vi "Periodic Tasks.vi"(8 "error in":errorcluster) -> ()   [LabVIEW 2017]
doc: "This VI runs in parallel to other tasks. It can contain as many user-defined periodic loops as you need. These can carry out PID or other sorts of timed response."
uses:
  <vilib>/Rock Robotics/WPI/ThirdParty/Phoenix-LabVIEW/Motor Controller/Controls/CTRE_Phoenix_MotorControl_ControlMode.ctl
  <vilib>/Rock Robotics/WPI/ThirdParty/Phoenix-LabVIEW/Motor Controller/Controls/CTRE_Phoenix_MotorControl_RemoteFeedbackDevice.ctl
  <vilib>/Rock Robotics/WPI/ThirdParty/Phoenix-LabVIEW/Motor Controller/Controls/CTRE_Phoenix_MotorControl_RemoteSourceType.ctl
  <vilib>/Rock Robotics/WPI/ThirdParty/Phoenix-LabVIEW/Controls/CTRE_Phoenix_Params.ctl
  <vilib>/Rock Robotics/WPI/Utilities/WPI_GetSetVariantRefNum.vi
panel:
  in  "Reverse Limit Threshold":i32
  in  "Forward Limit Threshold":i32
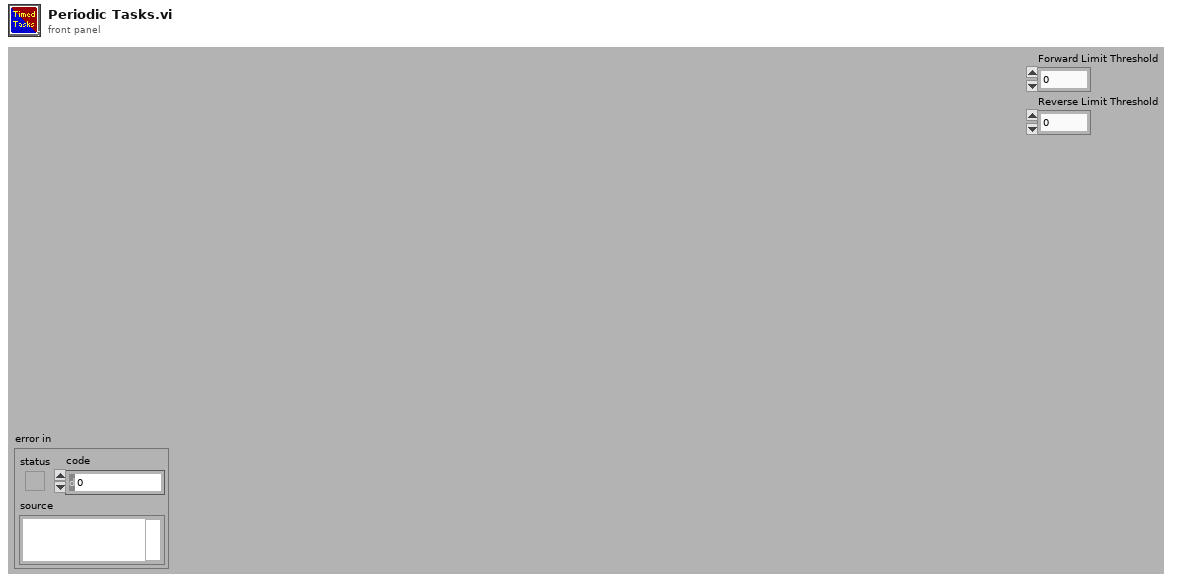
[diagram p1: front panel]
types:
  T1 = typedef "CTRE_PigeonIMU_DeviceRef.ctl" = cluster{"DeviceStatus":errorcluster, "Device Number":u8, "Type":T2, "Device ID":u32, "Handle":u64, "UsageFrame":u32, "Library Path":path}
  T2 = typedef "CTRE_PigeonIMU_ConnectionType.ctl" = u32
  T3 = typedef "CTRE_CANifier_DeviceRef.ctl" = cluster{"DeviceStatus":errorcluster, "Device Number":u8, "Handle":u64, "UsageFrame":u32, "Library Path":path}
  T4 = typedef "WPI_MotorControlDeviceRef.ctl" = cluster{"DeviceStatus":errorcluster, "Type":T5, "PWM":cluster{"PWM Channel":T6, "DeadBand":T7}, "CAN":cluster{"Device Number":u8, "SetOutput VI Ref":variant, "GetOutput VI Ref":variant, "Enable VI Ref":variant, "Disable VI Ref":variant, "Data":variant}, "Invert":bool, "DIO PWM":cluster{"PWM \"Enable\" Channel":T6, "DIOChannel":T8, "PWM Rate":dbl}}
  T5 = typedef "WPI_MotorControlType.ctl" = enum16{"PWM", "CAN", "DIO PWM"}
  T6 = typedef "FPGA_DIOPWMChannel.ctl" = enum8{"PWM 0", "PWM 1", "PWM 2", "PWM 3", "PWM 4", "PWM 5", "PWM 6", "PWM 7", "PWM 8", "PWM 9", "PWM MXP 0", "PWM MXP 1", "PWM MXP 2", "PWM MXP 3", "PWM MXP 4", "PWM MXP 5", "PWM MXP 6", "PWM MXP 7", "PWM MXP 8", "PWM MXP 9", "Invalid"}
  T7 = typedef "WPI_PWMDeadband.ctl" = cluster{"Name":string, "maxPositivePwm":i32, "minPositivePwm":i32, "centerPwm":i32, "maxNegativePwm":i32, "minNegativePwm":i32, "angularRange":u16}
  T8 = typedef "FPGA_DIOChannel.ctl" = enum8{"DIO 0", "DIO 1", "DIO 2", "DIO 3", "DIO 4", "DIO 5", "DIO 6", "DIO 7", "DIO 8", "DIO 9", "DIO MXP 0", "DIO MXP 1", "DIO MXP 2", "DIO MXP 3", "DIO MXP 4", "DIO MXP 5", "DIO MXP 6", "DIO MXP 7", "DIO MXP 8", "DIO MXP 9", "DIO MXP 10", "DIO MXP 11", "DIO MXP 12", "DIO MXP 13", "DIO MXP 14", "DIO MXP 15", "SPI Port CS1", "SPI Port CS2", "SPI Port CS3", "SPI Port MISO", "SPI Port MOSI", "Invalid"}
  T9 = typedef "WPI_JoystickDevRef.ctl" = cluster{"Device":T10}
  T10 = typedef "WPI_JoystickDeviceEnum.ctl" = enum16{"USB 0", "USB 1", "USB 2", "USB 3", "USB 4", "USB 5"}
  T11 = typedef "CTRE_Phoenix_MotorControl_RemoteSourceType.ctl" = enum16{"Off", "Talon SRX Selected Sensor", "Pigeon IMU Yaw", "Pigeon IMU Pitch", "Pigeon IMU Roll", "CANifier Quadrature", "CANifier PWM Input 0", "CANifier PWM Input 1", "CANifier PWM Input 2", "CANifier PWM Input 3"}
  T12 = typedef "CTRE_Phoenix_MotorControl_ControlMode.ctl" = u16
  T13 = typedef "CTRE_Phoenix_MotorControl_RemoteFeedbackDevice.ctl" = i8
  T14 = typedef "CTRE_Phoenix_Params.ctl" = u16
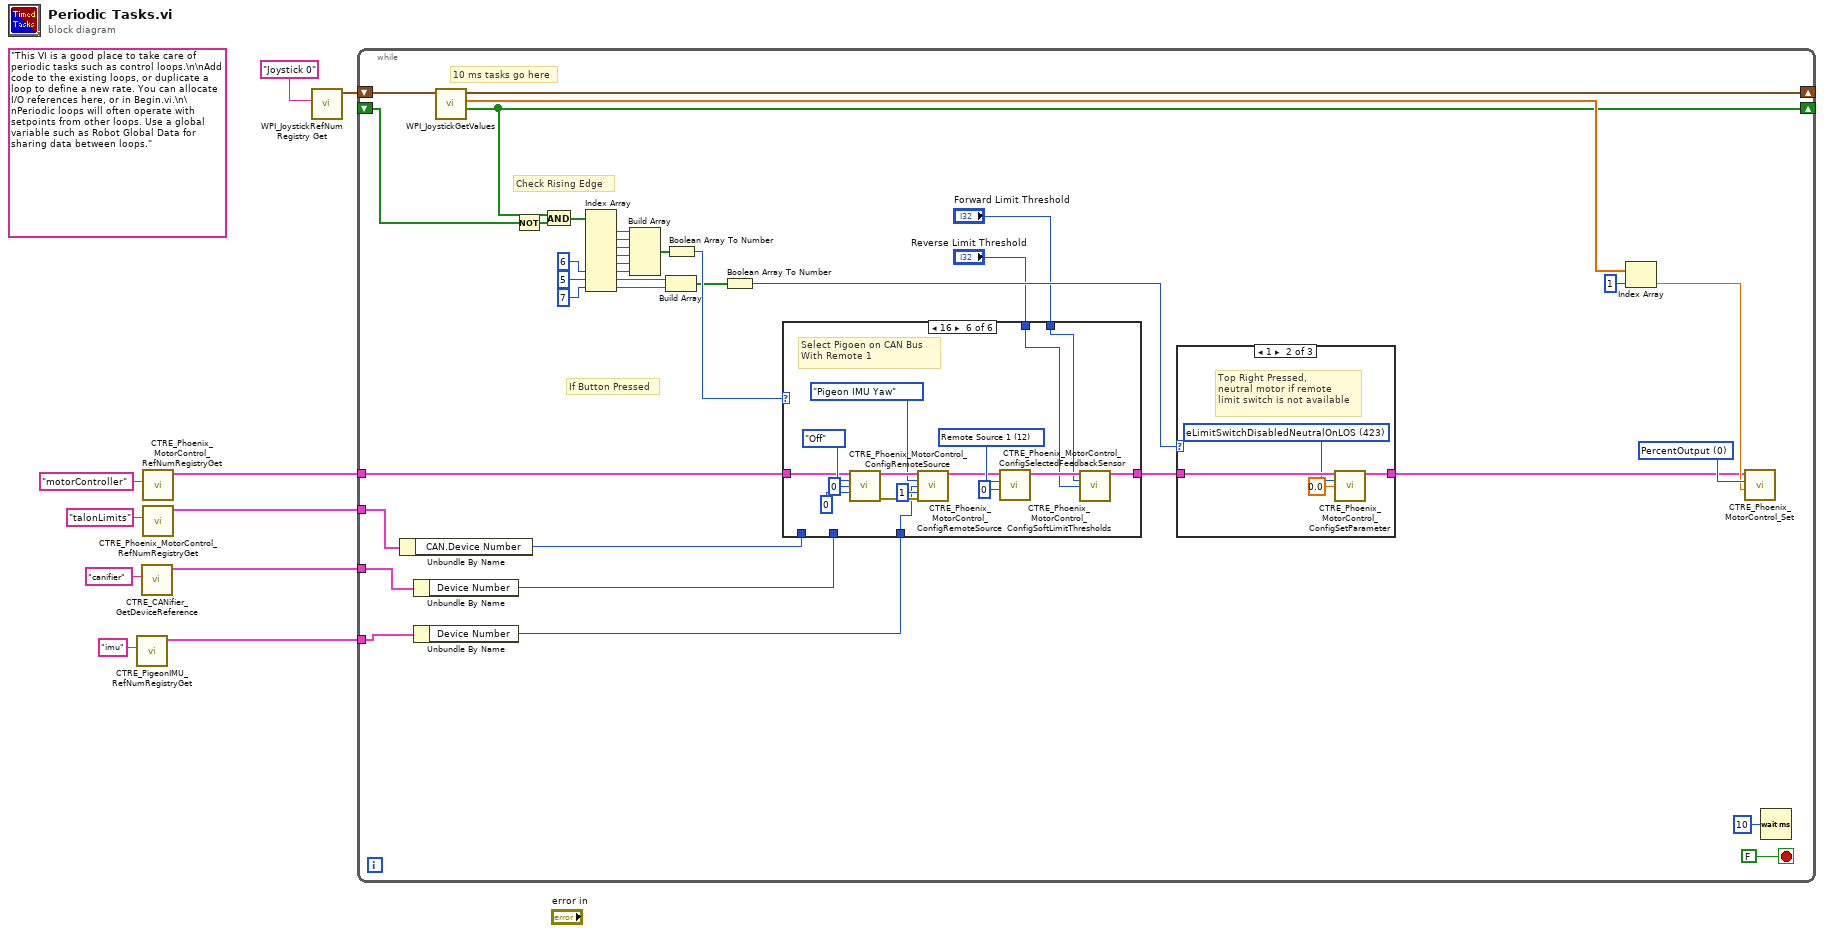
[diagram p0: block diagram]
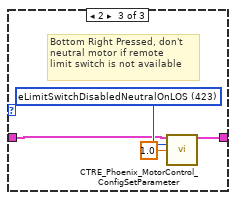
[diagram p3: hidden frame]
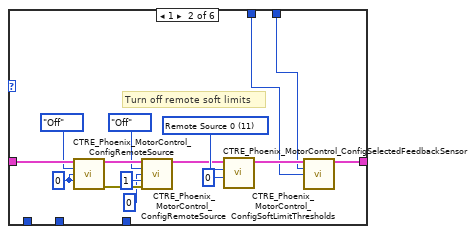
[diagram p5: hidden frame]
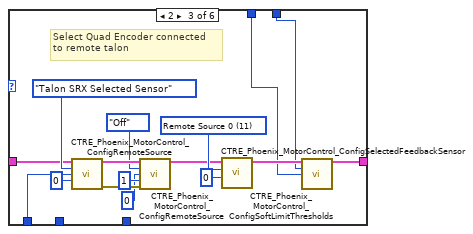
[diagram p6: hidden frame]
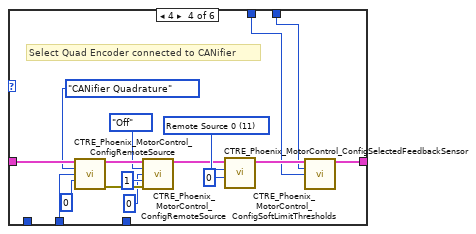
[diagram p7: hidden frame]
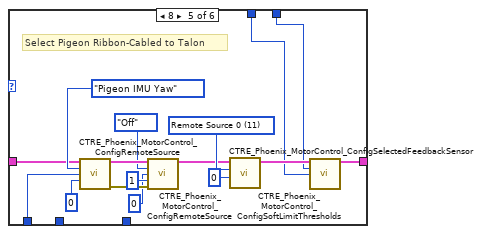
[diagram p8: hidden frame]
diagram:
  (unwired) "This VI is a good place to take care of periodic tasks such as control loops.\n\nAdd code to the existing loops, or duplicate a loop to define a new rate. You can allocate I/O references here, or in Begin.vi.\n\nPeriodic loops will often operate with setpoints from other loops. Use a global variable such as Robot Global Data for sharing data between loops."
  n1 = call <vilib>:"CTRE_PigeonIMU_RefNumRegistryGet.vi"("refnum name"="imu") -> ("PigeonIMUDevRef"=w1:T1)  [unwired: 9 in, 1 out]
  n2 = call <vilib>:"CTRE_CANifier_GetDeviceReference.vi"("refnum name"="canifier") -> ("CANifierDevRef"=w5:T3)  [unwired: 9 in, 1 out]
  n3 = call <vilib>:"CTRE_Phoenix_MotorControl_RefNumRegistryGet.vi"("refnum name"="motorController") -> ("PhoenixMotorControlDevRef"=w3:T4)  [unwired: 9 in, 1 out]
  n4 = call <vilib>:"CTRE_Phoenix_MotorControl_RefNumRegistryGet.vi"("refnum name"="talonLimits") -> ("PhoenixMotorControlDevRef"=w4:T4)  [unwired: 9 in, 1 out]
  n5 = call <vilib>:"WPI_JoystickRefNum Registry Get.vi"("refnum name"="Joystick 0") -> ("JoystickDevRef"=w9:T9)  [unwired: 1 in, 9 out]
  n6 = while {
    shift-right: [w44] -> _
    shift-left: w9 -> [w45]
    tunnel: w5 -> [w34]
    tunnel: w4 -> [w35]
    tunnel: w3 -> [w36]
    shift-right: [w39] -> _
    shift-left: _ -> [w40]
    tunnel: w1 -> [w12]
    stop <- FALSE stop-if-true
    w46 = T12 0 items=["PercentOutput"=0, "Position"=1, "Velocity"=2, "Current"=3, "Follower"=5, "MotionProfile"=6, "MotionMagic"=7, "MotionMagicArc"=8, "MotionProfileArc"=10, "Disabled"=15] ("Control Mode")
    # "If Button Pressed"
    # "Check Rising Edge"
    # "10 ms tasks go here"
    n7 = Unbundle By Name(w35) -> ("CAN.Device Number"=w27:u8)
    n8 = Unbundle By Name(w34) -> ("Device Number"=w26:u8)
    n9 = Unbundle By Name(w12) -> ("Device Number"=w11:u8)
    n10 = call <vilib>:"WPI_JoystickGetValues.vi"("JoystickDevRef"=w45) -> ("Buttons"=w39:bool[], "Axes"=w43:dbl[], "JoystickDevRef"=w44:T9)  [unwired: 6 in, 2 out]
    n11 = Not(x=w40) -> (.not. x?=w38:bool[])
    n12 = And(x=w39, y=w38) -> (x .and. y?=w37:bool[])
    n13 = Index Array(array=w37, index #6=6 ("index"), index #7=5 ("index"), index #8=7 ("index")) -> (element #1=w33:bool, element #2=w30:bool, element #3=w31:bool, element #4=w32:bool, element #5=w21:bool, element #6=w20:bool, element #7=w19:bool, element #8=w18:bool)  [unwired: 5 in]
    n14 = Build Array(w33, w30, w31, w32, w21, w20) -> (w29:bool[])
    n15 = Build Array(w19, w18) -> (w25:bool[])
    n16 = Boolean Array To Number(Boolean array=w29) -> (number=w28:u32)
    n17 = Boolean Array To Number(Boolean array=w25) -> (number=w23:u32)
    n18 = case shown="16" w28 {
      tunnel: w36 -> [w58 w72 w76 w95 w111 w127]
      tunnel: w27 -> [_ _ w80 _ w108 _]
      tunnel: w26 -> [_ _ _ w91 _ _]
      tunnel: [w58 w63 w75 w96 w112 w128] -> w22
      tunnel: "Reverse Limit Threshold" -> [_ w61 w78 w92 w110 w124]
      tunnel: "Forward Limit Threshold" -> [_ w62 w79 w93 w109 w125]
      tunnel: w11 -> [_ _ _ _ _ w126]
      frame 0, Default {
        # "Nothing pressed"
      }
      frame 1 {
        w59 = u32 0 ("Source Index (0/1)")
        w73 = T13 11 items=["None"=-1, "Sensor Sum (S0 + S1)"=9, "Sensor Difference (D0 - D1)"=10, "Remote Source 0"=11, "Remote Source 1"=12, "Software Emulated"=15] ("Feedback Device")
        # "Turn off remote soft limits"
        n19 = call <vilib>:"CTRE_Phoenix_MotorControl_ConfigRemoteSource.vi"("PhoenixMotorControlDevRef"=w72, "Remote Device Type"=CTRE_Phoenix_MotorControl_RemoteSourceType."Off", "Remote Device ID"=w59, "Source Index (0/1)"=w59) -> ("PhoenixMotorControlDevRef"=w69:T4, "error out"=w68:errorcluster)  [unwired: 10 in]
        n20 = call <vilib>:"CTRE_Phoenix_MotorControl_ConfigRemoteSource.vi"("PhoenixMotorControlDevRef"=w69, "Remote Device Type"=CTRE_Phoenix_MotorControl_RemoteSourceType."Off", "Remote Device ID"=u8 0, "Source Index (0/1)"=u32 1, "error in (no error)"=w68) -> ("PhoenixMotorControlDevRef"=w66:T4)  [unwired: 9 in, 1 out]
        n21 = call <vilib>:"CTRE_Phoenix_MotorControl_ConfigSelectedFeedbackSensor.vi"("pidLoopIdx"=0, "Feedback Device"=w73, "PhoenixMotorControlDevRef"=w66) -> ("PhoenixMotorControlDevRef"=w64:T4)  [unwired: 7 in, 1 out]
        n22 = call <vilib>:"CTRE_Phoenix_MotorControl_ConfigSoftLimitThresholds.vi"("PhoenixMotorControlDevRef"=w64, "Forward Soft Limit"=w62, "Reverse Soft Limit"=w61) -> ("PhoenixMotorControlDevRef"=w63:T4)  [unwired: 11 in, 1 out]
      }
      frame 2 {
        w89 = T13 11 items=["None"=-1, "Sensor Sum (S0 + S1)"=9, "Sensor Difference (D0 - D1)"=10, "Remote Source 0"=11, "Remote Source 1"=12, "Software Emulated"=15] ("Feedback Device")
        # "Select Quad Encoder connected\nto remote talon"
        n23 = call <vilib>:"CTRE_Phoenix_MotorControl_ConfigRemoteSource.vi"("PhoenixMotorControlDevRef"=w76, "Remote Device Type"=CTRE_Phoenix_MotorControl_RemoteSourceType."Talon SRX Selected Sensor", "Remote Device ID"=w80, "Source Index (0/1)"=u32 0) -> ("PhoenixMotorControlDevRef"=w86:T4, "error out"=w85:errorcluster)  [unwired: 10 in]
        n24 = call <vilib>:"CTRE_Phoenix_MotorControl_ConfigRemoteSource.vi"("PhoenixMotorControlDevRef"=w86, "Remote Device Type"=CTRE_Phoenix_MotorControl_RemoteSourceType."Off", "Remote Device ID"=u8 0, "Source Index (0/1)"=u32 1, "error in (no error)"=w85) -> ("PhoenixMotorControlDevRef"=w83:T4)  [unwired: 9 in, 1 out]
        n25 = call <vilib>:"CTRE_Phoenix_MotorControl_ConfigSelectedFeedbackSensor.vi"("pidLoopIdx"=0, "Feedback Device"=w89, "PhoenixMotorControlDevRef"=w83) -> ("PhoenixMotorControlDevRef"=w81:T4)  [unwired: 7 in, 1 out]
        n26 = call <vilib>:"CTRE_Phoenix_MotorControl_ConfigSoftLimitThresholds.vi"("PhoenixMotorControlDevRef"=w81, "Forward Soft Limit"=w79, "Reverse Soft Limit"=w78) -> ("PhoenixMotorControlDevRef"=w75:T4)  [unwired: 11 in, 1 out]
      }
      frame 4 {
        w105 = T13 11 items=["None"=-1, "Sensor Sum (S0 + S1)"=9, "Sensor Difference (D0 - D1)"=10, "Remote Source 0"=11, "Remote Source 1"=12, "Software Emulated"=15] ("Feedback Device")
        # "Select Quad Encoder connected to CANifier"
        n27 = call <vilib>:"CTRE_Phoenix_MotorControl_ConfigRemoteSource.vi"("PhoenixMotorControlDevRef"=w95, "Remote Device Type"=CTRE_Phoenix_MotorControl_RemoteSourceType."CANifier Quadrature", "Remote Device ID"=w91, "Source Index (0/1)"=u32 0) -> ("PhoenixMotorControlDevRef"=w103:T4, "error out"=w102:errorcluster)  [unwired: 10 in]
        n28 = call <vilib>:"CTRE_Phoenix_MotorControl_ConfigRemoteSource.vi"("PhoenixMotorControlDevRef"=w103, "Remote Device Type"=CTRE_Phoenix_MotorControl_RemoteSourceType."Off", "Remote Device ID"=u8 0, "Source Index (0/1)"=u32 1, "error in (no error)"=w102) -> ("PhoenixMotorControlDevRef"=w100:T4)  [unwired: 9 in, 1 out]
        n29 = call <vilib>:"CTRE_Phoenix_MotorControl_ConfigSelectedFeedbackSensor.vi"("pidLoopIdx"=0, "Feedback Device"=w105, "PhoenixMotorControlDevRef"=w100) -> ("PhoenixMotorControlDevRef"=w98:T4)  [unwired: 7 in, 1 out]
        n30 = call <vilib>:"CTRE_Phoenix_MotorControl_ConfigSoftLimitThresholds.vi"("PhoenixMotorControlDevRef"=w98, "Forward Soft Limit"=w93, "Reverse Soft Limit"=w92) -> ("PhoenixMotorControlDevRef"=w96:T4)  [unwired: 11 in, 1 out]
      }
      frame 8 {
        w121 = T13 11 items=["None"=-1, "Sensor Sum (S0 + S1)"=9, "Sensor Difference (D0 - D1)"=10, "Remote Source 0"=11, "Remote Source 1"=12, "Software Emulated"=15] ("Feedback Device")
        # "Select Pigeon Ribbon-Cabled to Talon"
        n31 = call <vilib>:"CTRE_Phoenix_MotorControl_ConfigRemoteSource.vi"("PhoenixMotorControlDevRef"=w111, "Remote Device Type"=CTRE_Phoenix_MotorControl_RemoteSourceType."Pigeon IMU Yaw", "Remote Device ID"=w108, "Source Index (0/1)"=u32 0) -> ("PhoenixMotorControlDevRef"=w119:T4, "error out"=w118:errorcluster)  [unwired: 10 in]
        n32 = call <vilib>:"CTRE_Phoenix_MotorControl_ConfigRemoteSource.vi"("PhoenixMotorControlDevRef"=w119, "Remote Device Type"=CTRE_Phoenix_MotorControl_RemoteSourceType."Off", "Remote Device ID"=u8 0, "Source Index (0/1)"=u32 1, "error in (no error)"=w118) -> ("PhoenixMotorControlDevRef"=w116:T4)  [unwired: 9 in, 1 out]
        n33 = call <vilib>:"CTRE_Phoenix_MotorControl_ConfigSelectedFeedbackSensor.vi"("pidLoopIdx"=0, "Feedback Device"=w121, "PhoenixMotorControlDevRef"=w116) -> ("PhoenixMotorControlDevRef"=w114:T4)  [unwired: 7 in, 1 out]
        n34 = call <vilib>:"CTRE_Phoenix_MotorControl_ConfigSoftLimitThresholds.vi"("PhoenixMotorControlDevRef"=w114, "Forward Soft Limit"=w109, "Reverse Soft Limit"=w110) -> ("PhoenixMotorControlDevRef"=w112:T4)  [unwired: 11 in, 1 out]
      }
      frame 16 {
        w137 = T13 12 items=["None"=-1, "Sensor Sum (S0 + S1)"=9, "Sensor Difference (D0 - D1)"=10, "Remote Source 0"=11, "Remote Source 1"=12, "Software Emulated"=15] ("Feedback Device")
        # "Select Pigoen on CAN Bus\nWith Remote 1"
        n35 = call <vilib>:"CTRE_Phoenix_MotorControl_ConfigRemoteSource.vi"("PhoenixMotorControlDevRef"=w127, "Remote Device Type"=CTRE_Phoenix_MotorControl_RemoteSourceType."Off", "Remote Device ID"=u8 0, "Source Index (0/1)"=u32 0) -> ("PhoenixMotorControlDevRef"=w135:T4, "error out"=w134:errorcluster)  [unwired: 10 in]
        n36 = call <vilib>:"CTRE_Phoenix_MotorControl_ConfigRemoteSource.vi"("PhoenixMotorControlDevRef"=w135, "Remote Device Type"=CTRE_Phoenix_MotorControl_RemoteSourceType."Pigeon IMU Yaw", "Remote Device ID"=w126, "Source Index (0/1)"=u32 1, "error in (no error)"=w134) -> ("PhoenixMotorControlDevRef"=w132:T4)  [unwired: 9 in, 1 out]
        n37 = call <vilib>:"CTRE_Phoenix_MotorControl_ConfigSelectedFeedbackSensor.vi"("pidLoopIdx"=0, "Feedback Device"=w137, "PhoenixMotorControlDevRef"=w132) -> ("PhoenixMotorControlDevRef"=w130:T4)  [unwired: 7 in, 1 out]
        n38 = call <vilib>:"CTRE_Phoenix_MotorControl_ConfigSoftLimitThresholds.vi"("PhoenixMotorControlDevRef"=w130, "Forward Soft Limit"=w125, "Reverse Soft Limit"=w124) -> ("PhoenixMotorControlDevRef"=w128:T4)  [unwired: 11 in, 1 out]
      }
    }
    n39 = case shown="1" w23 {
      tunnel: [w49 w53 w55] -> w24
      tunnel: w22 -> [w49 w52 w54]
      frame 0, Default {
      }
      frame 1 {
        w51 = T14 423 items=["eOnBoot_BrakeMode"=31, "eQuadFilterEn"=91, "eQuadIdxPolarity"=108, "eClearPositionOnIdx"=100, "eMotionProfileHasUnderrunErr"=119, "eMotionProfileTrajectoryPointDurationMs"=120, "eClearPosOnLimitF"=144, "eClearPosOnLimitR"=145, "eStatusFramePeriod"=300, "eOpenLoopRamp"=301, "eClosedLoopRamp"=302, "eNeutralDeadband"=303, "ePeakPosOutput"=305, "eNominalPosOutput"=306, "ePeakNegOutput"=307, "eNominalNegOutput"=308, "eProfileParamSlot_P"=310, "eProfileParamSlot_I"=311, "eProfileParamSlot_D"=312, "eProfileParamSlot_F"=313, "eProfileParamSlot_IZone"=314, "eProfileParamSlot_AllowableErr"=315, "eProfileParamSlot_MaxIAccum"=316, "eClearPositionOnLimitF"=320, "eClearPositionOnLimitR"=321, "eClearPositionOnQuadIdx"=322, "eSampleVelocityPeriod"=325, "eSampleVelocityWindow"=326, "eFeedbackSensorType"=330, "eSelectedSensorPosition"=331, "eFeedbackNotContinuous"=332, "eRemoteSensorSource"=333, "eRemoteSensorDeviceID"=334, "eSensorTerm"=335, "eRemoteSensorClosedLoopDisableNeutralOnLOS"=336, "eForwardSoftLimitThreshold"=340, "eReverseSoftLimitThreshold"=341, "eForwardSoftLimitEnable"=342, "eReverseSoftLimitEnable"=343, "eNominalBatteryVoltage"=350, "eBatterVoltageFilterSize"=351, "eContinuousCurrentLimitAmps"=360, "eContinuousCurrentLimitMs"=361, "ePeakCurrentLimitAmps"=362, "eClosedLoopIAccum"=370, "eCustomParam"=380, "eStickyFaults"=390, "eAnalogPosition"=400, "eQuadraturePosition"=401, "ePulseWidthPosition"=402, "eMotMag_Accel"=410, "eMotMag_VelCruise"=411, "eLimitSwitchSource"=421, "eLimitSwitchNormClosedAndDis"=422, "eLimitSwitchDisabledNeutralOnLOS"=423, "eLimitSwitchRemoteDevID"=424] ("Parameter")
        # "Top Right Pressed,\nneutral motor if remote\nlimit switch is not available"
        n40 = call <vilib>:"CTRE_Phoenix_MotorControl_ConfigSetParameter.vi"("PhoenixMotorControlDevRef"=w52, "Parameter"=w51, "value"=0.0) -> ("PhoenixMotorControlDevRef"=w53:T4)  [unwired: 11 in, 1 out]
      }
      frame 2 {
        w57 = T14 423 items=["eOnBoot_BrakeMode"=31, "eQuadFilterEn"=91, "eQuadIdxPolarity"=108, "eClearPositionOnIdx"=100, "eMotionProfileHasUnderrunErr"=119, "eMotionProfileTrajectoryPointDurationMs"=120, "eClearPosOnLimitF"=144, "eClearPosOnLimitR"=145, "eStatusFramePeriod"=300, "eOpenLoopRamp"=301, "eClosedLoopRamp"=302, "eNeutralDeadband"=303, "ePeakPosOutput"=305, "eNominalPosOutput"=306, "ePeakNegOutput"=307, "eNominalNegOutput"=308, "eProfileParamSlot_P"=310, "eProfileParamSlot_I"=311, "eProfileParamSlot_D"=312, "eProfileParamSlot_F"=313, "eProfileParamSlot_IZone"=314, "eProfileParamSlot_AllowableErr"=315, "eProfileParamSlot_MaxIAccum"=316, "eClearPositionOnLimitF"=320, "eClearPositionOnLimitR"=321, "eClearPositionOnQuadIdx"=322, "eSampleVelocityPeriod"=325, "eSampleVelocityWindow"=326, "eFeedbackSensorType"=330, "eSelectedSensorPosition"=331, "eFeedbackNotContinuous"=332, "eRemoteSensorSource"=333, "eRemoteSensorDeviceID"=334, "eSensorTerm"=335, "eRemoteSensorClosedLoopDisableNeutralOnLOS"=336, "eForwardSoftLimitThreshold"=340, "eReverseSoftLimitThreshold"=341, "eForwardSoftLimitEnable"=342, "eReverseSoftLimitEnable"=343, "eNominalBatteryVoltage"=350, "eBatterVoltageFilterSize"=351, "eContinuousCurrentLimitAmps"=360, "eContinuousCurrentLimitMs"=361, "ePeakCurrentLimitAmps"=362, "eClosedLoopIAccum"=370, "eCustomParam"=380, "eStickyFaults"=390, "eAnalogPosition"=400, "eQuadraturePosition"=401, "ePulseWidthPosition"=402, "eMotMag_Accel"=410, "eMotMag_VelCruise"=411, "eLimitSwitchSource"=421, "eLimitSwitchNormClosedAndDis"=422, "eLimitSwitchDisabledNeutralOnLOS"=423, "eLimitSwitchRemoteDevID"=424] ("Parameter")
        # "Bottom Right Pressed, don't\nneutral motor if remote\nlimit switch is not available"
        n41 = call <vilib>:"CTRE_Phoenix_MotorControl_ConfigSetParameter.vi"("PhoenixMotorControlDevRef"=w54, "Parameter"=w57, "value"=1.0) -> ("PhoenixMotorControlDevRef"=w55:T4)  [unwired: 11 in, 1 out]
      }
    }
    n42 = Index Array(array=w43, index=1) -> (element=w41:dbl)
    n43 = call <vilib>:"CTRE_Phoenix_MotorControl_Set.vi"("Output"=w41, "Control Mode"=w46, "PhoenixMotorControlDevRef"=w24) -> ()  [unwired: 7 in, 2 out]
    n44 = Wait (ms)(milliseconds to wait=u32 10) -> ()  [unwired: 1 out]
  }
